vi "saveToCSV_a_funcionar.vi"() -> ()   [LabVIEW 2018]
uses:
  <vilib>/Utility/file.llb/Write Delimited Spreadsheet (string).vi
panel:
  out "Iteration":i32
  in  "stop":bool
  out "Temperature":dbl
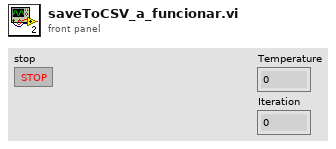
[diagram p1: front panel]
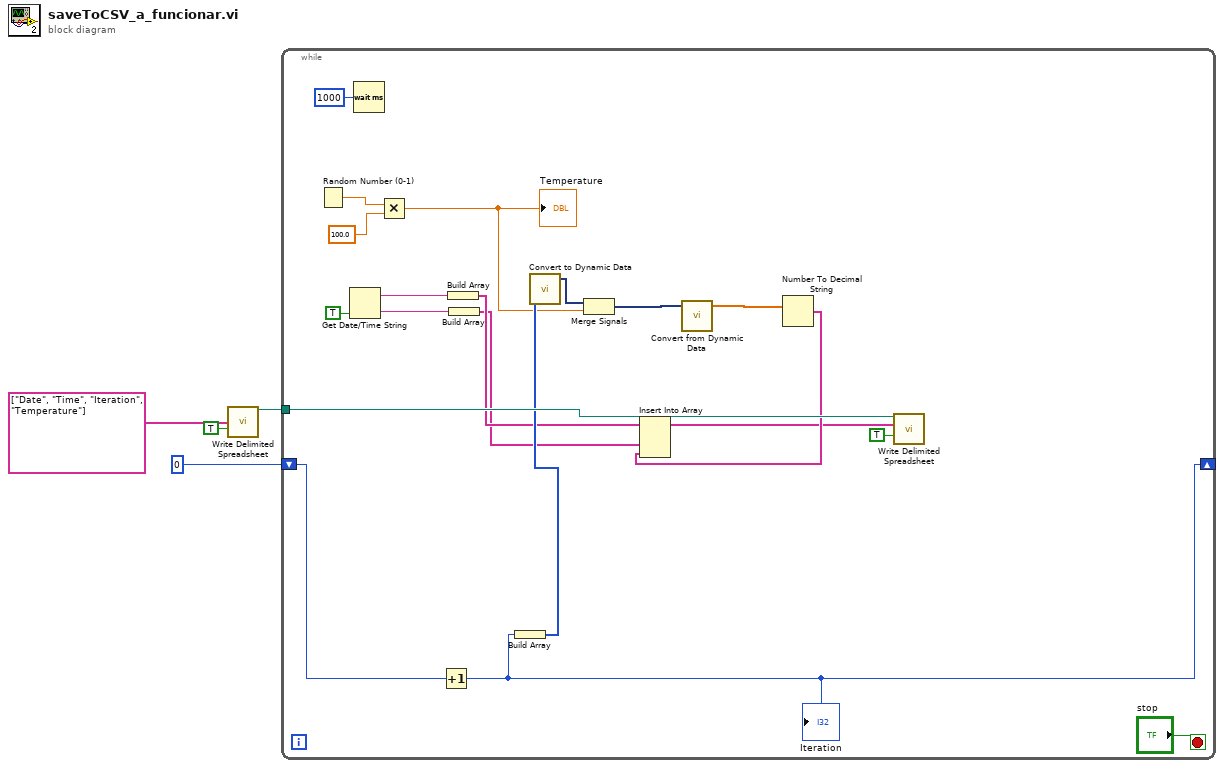
[diagram p0: block diagram]
diagram:
  n1 = call-poly <vilib>:"Write Delimited Spreadsheet.vi"("1D data"=string[] ["Date", "Time", "Iteration", "Temperature"], "append to file? (new file:F)"=TRUE) -> ("new file path (Not A Path if cancelled)"=w2:path)  [unwired: 12 in, 1 out]
  n2 = while {
    shift-right: [w16] -> _
    shift-left: 0 -> [w20]
    tunnel: w2 -> [w19]
    stop <- "stop" stop-if-true
    n3 = Random Number (0-1)() -> (number: 0 to 1=w22:dbl)
    n4 = Get Date/Time String(want seconds? (F)=TRUE) -> (date string=w18:string, time string=w17:string)  [unwired: 2 in]
    n5 = Wait (ms)(milliseconds to wait=u32 1000) -> ()  [unwired: 1 out]
    n6 = Multiply(x=w22, y=100.0) -> (x*y=w13:dbl)
    "Temperature" <- w13
    n7 = Increment(x=w20) -> (x+1=w16:i32)
    "Iteration" <- w16
    n8 = Build Array(w18) -> (w10:string[])
    n9 = Build Array(w17) -> (w9:string[])
    n10 = Build Array(w16) -> (w15:i32[])
    n11 = call "Convert to Dynamic Data"("Array"=w15) -> ("Dynamic Data Type"=w14:dynamicdata)  [unwired: 3 in]
    n12 = Merge Signals(w14, w13) -> (w12:dynamicdata)
    n13 = call "Convert from Dynamic Data"("Dynamic Data Type"=w12) -> ("Array"=w11:dbl[])  [unwired: 3 in]
    n14 = Number To Decimal String(number=w11) -> (decimal integer string=w8:string[])  [unwired: 1 in]
    n15 = Insert Into Array(array=w10, new element #1=w9, new element #2=w8) -> (w7:string[])  [unwired: 1 in]
    n16 = call-poly <vilib>:"Write Delimited Spreadsheet.vi"("file path (dialog if empty)"=w19, "1D data"=w7, "append to file? (new file:F)"=TRUE) -> ()  [unwired: 11 in, 2 out]
  }
